vi "TestCommandSerial.vi"(8 "error in (no error)":errorcluster, 10 "baud rate (9600)":u32=9600, 11 "VISA resource name":refnum<visa-resource-name>="COM1") -> (0 "error out":errorcluster)   [LabVIEW 2014]
uses:
  <vilib>/Instr/_visa.llb/VISA Configure Serial Port (Instr).vi
panel:
  out "read buffer":string
  in  "write buffer":string
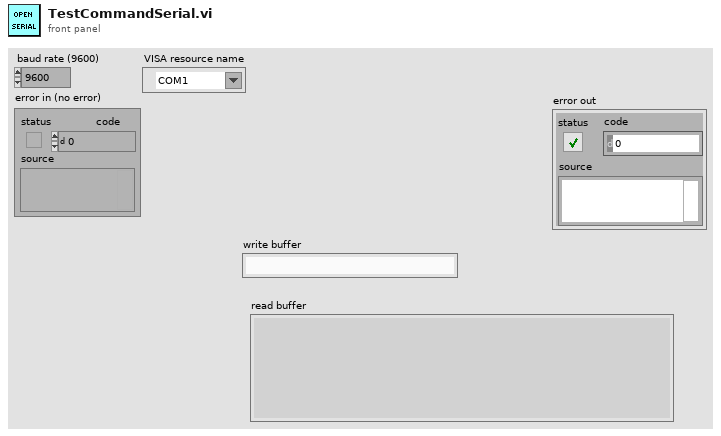
[diagram p1: front panel]
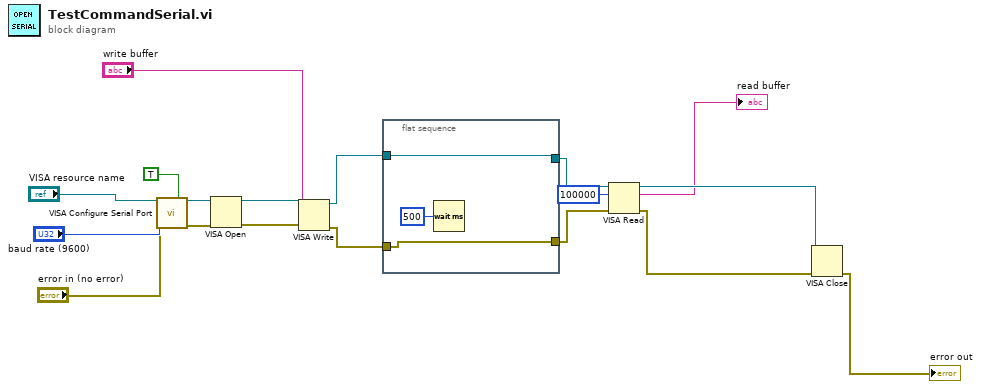
[diagram p0: block diagram]
diagram:
  n1 = call-poly "VISA Configure Serial Port"("VISA resource name"="VISA resource name", "Enable Termination\nChar (T)"=TRUE ("Enable Termination\nChar (T)"), "baud rate (9600)"="baud rate (9600)", "error in (no error)"="error in (no error)") -> ("VISA resource name out"=w17:refnum<visa-resource-name>, "error out"=w14:errorcluster)  [unwired: 10 in]
  n2 = VISA Open(error in (no error)=w14, VISA resource name=w17) -> (VISA resource name=w13:refnum<visa-resource-name>, error out=w11:errorcluster)  [unwired: 3 in]
  n3 = VISA Write(VISA resource name=w13, write buffer="write buffer", error in (no error)=w11) -> (VISA resource name out=w8:refnum<visa-resource-name>, error out=w7:errorcluster)  [unwired: 1 out]
  n4 = flat-sequence {
    tunnel: w8 -> [w20]
    tunnel: [w20] -> w6
    tunnel: w7 -> [w19]
    tunnel: [w19] -> w5
    frame #0 {
      n5 = Wait (ms)(milliseconds to wait=u32 500) -> ()  [unwired: 1 out]
    }
  }
  n6 = VISA Read(VISA resource name=w6, byte count=u32 100000, error in (no error)=w5) -> (VISA resource name out=w4:refnum<visa-resource-name>, read buffer=→"read buffer":string, error out=w3:errorcluster)  [unwired: 1 out]
  n7 = VISA Close(VISA resource name=w4, error in (no error)=w3) -> (error out=→"error out":errorcluster)
